vi "sensors.vi"() -> ()   [LabVIEW 2019]
doc: "This global variable contains sensor readings"
panel:
  out "CAN_Bus_Fault":bool
  out "Swerve_3_Actual_Shifter_State":bool
  out "Pose_Loop_Time (ms)":u32
  out "LIDAR_Distance_To_Target (in)":dbl
  out "Fused_Heading_To_Target (deg)":dbl
  out "LIDAR_Range_Valid":bool
  out "LimeLight_Range_Valid":bool
  out "LimeLight_PnP_Valid":bool
  out "Balls_Shot_Current":i32
  out "Control_Latency_Alarm":bool
  out "Battery_Critical":bool
  out "Electrical_Fault":bool
  out "Retrieved_Kicker_Power":dbl
  out "Time_Since_Pose_Update (ms)":u32
  out "Set_Robot_Pos":bool
  out "Set_Robot_Y (in)":dbl
  out "Set_Robot_X (in)":dbl
  out "Balls_Shot":i32
  out "Fused_Heading_To_Target_Delta (deg)":dbl
  out "In_Turret_Deadzone":bool
  out "IMU_Failure":bool
  out "Turret_Limit_Switch_B":bool
  out "Turret_Limit_Switch_A":bool
  out "Turret_Azimuth_Failure":bool
  out "Turret_Azimuth (deg)":dbl
  out "Turret_H (deg)":dbl
  out "Intake_Overheat":bool
  out "Intake_Temp (C)":u8
  out "Kicker_Temp (C)":u8
  out "Kicker_Speed (rpm)":dbl
  out "Shooter_Motor_Failure":bool[](array[boolean])
  out "Pointed_At_Target":bool
  out "Fused_Distance_To_Target (in)":dbl
  out "Swerve_2_Drive_Velocity (ft/s)":dbl
  out "Swerve_3_Drive_Velocity (ft/s)":dbl
  out "Swerve_1_Drive_Velocity (ft/s)":dbl
  out "Swerve_0_Drive_Velocity (ft/s)":dbl
  out "Retrieved_Shooter_Power":dbl
  out "Shooter_Overheat":bool[](array[boolean])
  out "Shooter_1_Temp (C)":u8
  out "Shooter_0_Temp (C)":u8
  out "Shooter_1_Speed (rpm)":dbl
  out "Shooter_0_Speed (rpm)":dbl
  out "Pressure_Leak":bool
  out "Swerve_Drive_Overheat":bool[](array[boolean])
  out "Swerve_Azimuth_Fault":bool[](array[boolean])
  out "Compressor_On":bool
  out "Pressure_Transducer (PSI)":dbl
  out "Control_Loop_Time (ms)":u32
  out "LimeLight_Valid":bool
  out "Battery_Voltage (V)":dbl
  out "Swerve_2_Drive_Temp (C)":u8
  out "Swerve_3_Drive_Temp (C)":u8
  out "Swerve_1_Drive_Temp (C)":u8
  out "Swerve_0_Drive_Temp (C)":u8
  out "Swerve_3_Azimuth_Position (deg)":dbl
  out "Swerve_2_Azimuth_Position (deg)":dbl
  out "Swerve_1_Azimuth_Position (deg)":dbl
  out "Swerve_0_Azimuth_Position (deg)":dbl
  out "Robot_H (deg)":dbl
  out "Push_Robot_H (deg)":dbl
  out "Push_Robot_Pos":bool
  out "Push_Robot_Y (in)":dbl
  out "Push_Robot_X (in)":dbl
  out "Robot_Y (in)":dbl
  out "Robot_X (in)":dbl
  # "--robot pose--"
  # "--power and electrical  management--"
  # "--compute resources--"
  # "--drive subsystem--"
  # "--intake and magazine subsystem--"
  # "--targeting info--"
  # "--pressure management--"
  # "--shooter subsystem--"
  # "--turret subsystem--"
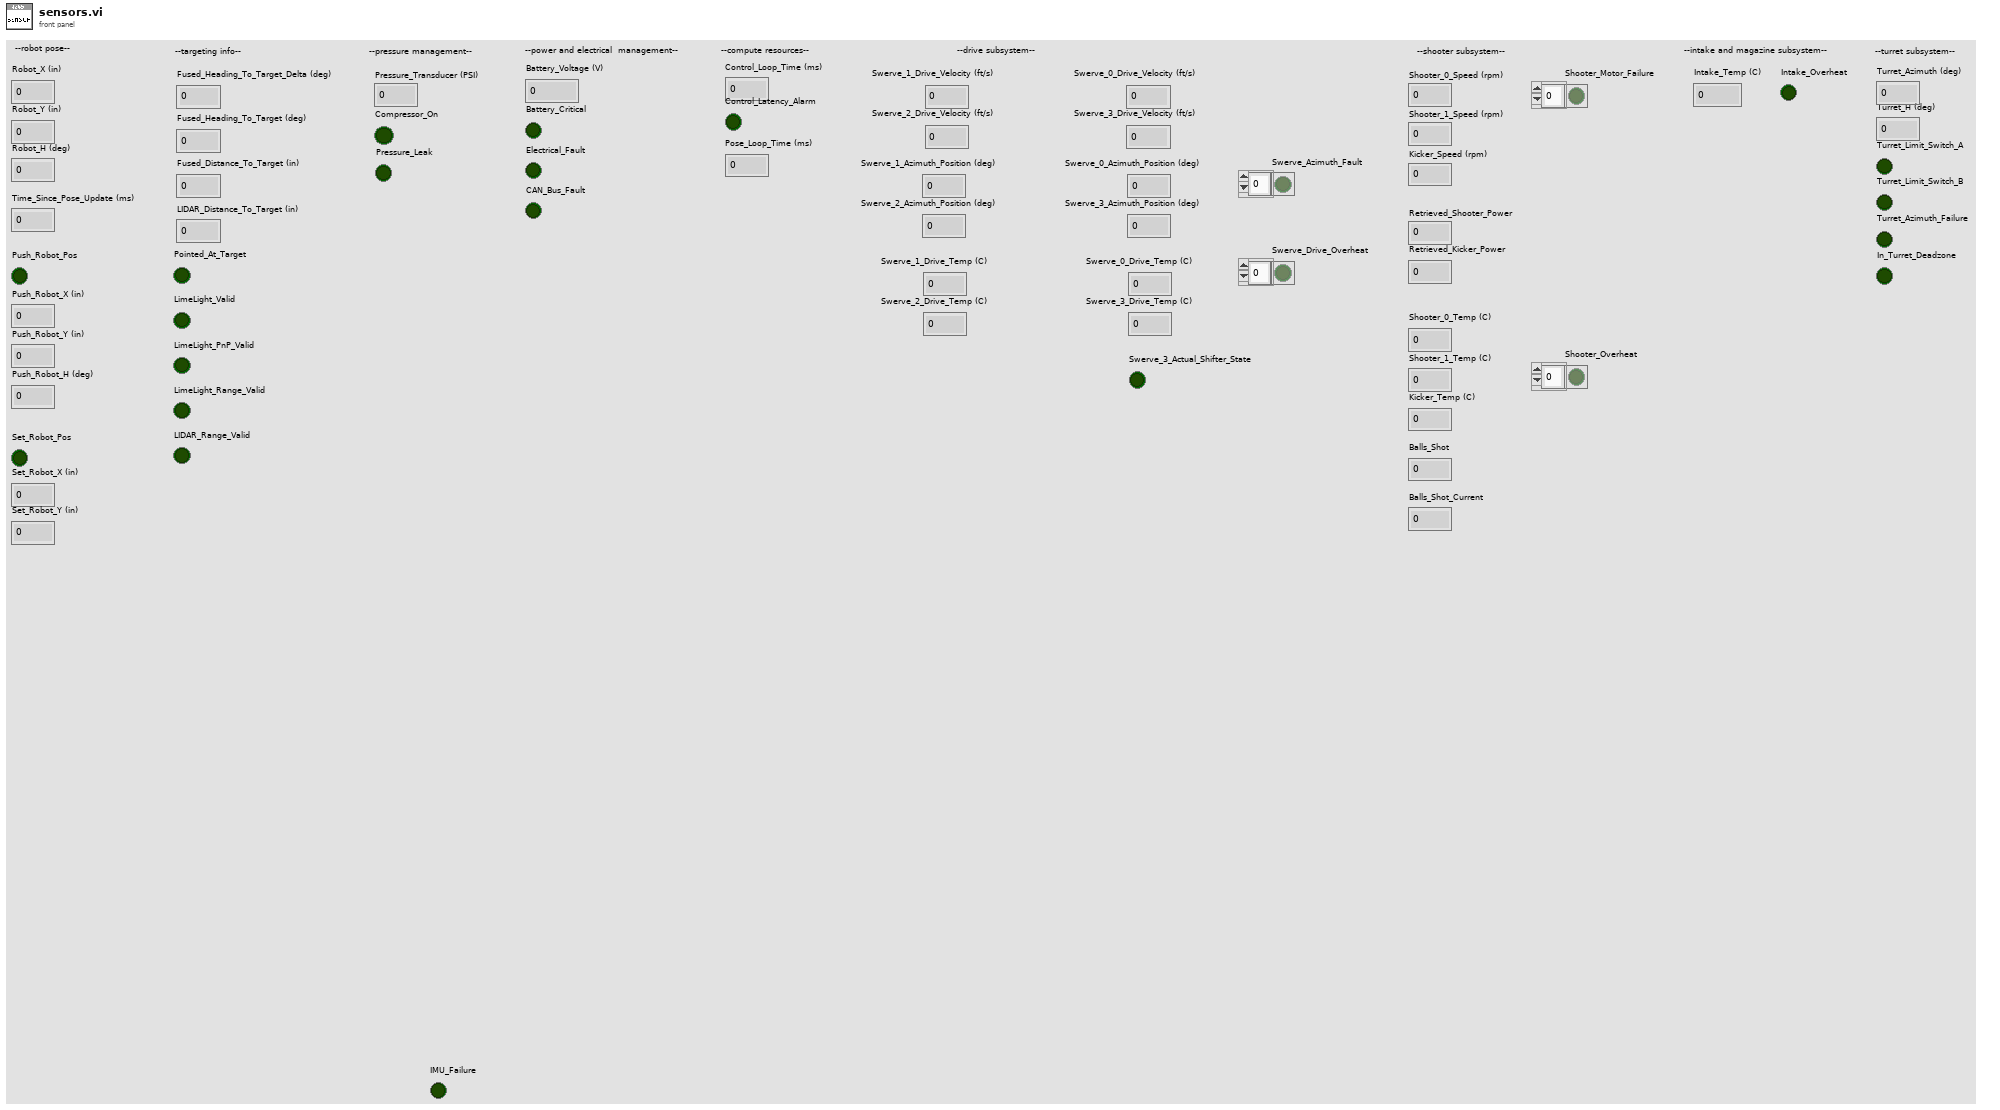
[diagram p1: front panel]
diagram:
